vi "sub_saveData.vi"(8 "에러 입력(에러 없음)":errorcluster, 9 "파일명":string, 10 "저장경로":path, 11 "VISA 참조 번호 입력":refnum<visa-resource-name>) -> (0 "에러 출력":errorcluster, 3 "VISA 참조 번호 출력":refnum<visa-resource-name>)   [LabVIEW 2020]
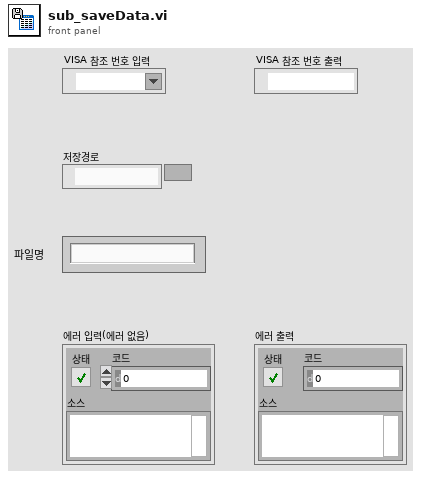
[diagram p1: front panel]
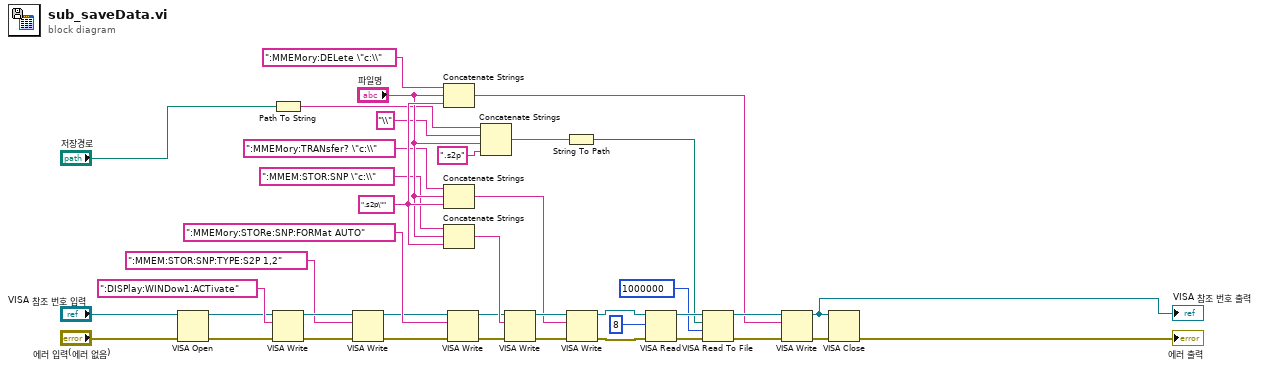
[diagram p0: block diagram]
diagram:
  w39 = ".s2p\"" ("문자열")
  n1 = VISA Open(error in (no error)="에러 입력(에러 없음)", VISA resource name="VISA 참조 번호 입력") -> (VISA resource name=w22:refnum<visa-resource-name>, error out=w23:errorcluster)  [unwired: 3 in]
  n2 = Path To String(path="저장경로") -> (string=w8:string)
  n3 = VISA Write(VISA resource name=w22, write buffer=":DISPlay:WINDow1:ACTivate" ("버퍼 쓰기"), error in (no error)=w23) -> (VISA resource name out=w24:refnum<visa-resource-name>, error out=w25:errorcluster)  [unwired: 1 out]
  n4 = VISA Write(VISA resource name=w24, write buffer=":MMEM:STOR:SNP:TYPE:S2P 1,2" ("버퍼 쓰기"), error in (no error)=w25) -> (VISA resource name out=w27:refnum<visa-resource-name>, error out=w28:errorcluster)  [unwired: 1 out]
  n5 = Concatenate Strings(":MMEMory:DELete \"c:\\" ("버퍼 쓰기"), "파일명", w39) -> (w3:string)
  n6 = Concatenate Strings(":MMEMory:TRANsfer? \"c:\\" ("버퍼 쓰기"), "파일명", w39) -> (w10:string)
  n7 = Concatenate Strings(":MMEM:STOR:SNP \"c:\\" ("버퍼 쓰기"), "파일명", w39) -> (w38:string)
  n8 = VISA Write(VISA resource name=w27, write buffer=":MMEMory:STORe:SNP:FORMat AUTO" ("버퍼 쓰기"), error in (no error)=w28) -> (VISA resource name out=w30:refnum<visa-resource-name>, error out=w34:errorcluster)  [unwired: 1 out]
  n9 = Concatenate Strings(w8, "\\" ("문자열"), "파일명", ".s2p" ("문자열")) -> (w7:string)
  n10 = VISA Write(VISA resource name=w30, write buffer=w38, error in (no error)=w34) -> (VISA resource name out=w31:refnum<visa-resource-name>, error out=w35:errorcluster)  [unwired: 1 out]
  n11 = String To Path(string=w7) -> (path=w6:path)
  n12 = VISA Write(VISA resource name=w31, write buffer=w10, error in (no error)=w35) -> (VISA resource name out=w33:refnum<visa-resource-name>, error out=w11:errorcluster)  [unwired: 1 out]
  n13 = VISA Read(VISA resource name=w33, byte count=u32 8 ("바이트 카운트"), error in (no error)=w11) -> (VISA resource name out=w32:refnum<visa-resource-name>, error out=w9:errorcluster)  [unwired: 2 out]
  n14 = VISA Read To File(8:w9, 9:u32 1000000 ("바이트 카운트"), 10:w6, 11:w32) -> (0:w4:errorcluster, 3:w5:refnum<visa-resource-name>)  [unwired: 1 out]
  n15 = VISA Write(VISA resource name=w5, write buffer=w3, error in (no error)=w4) -> (VISA resource name out=w40:refnum<visa-resource-name>, error out=w2:errorcluster)  [unwired: 1 out]
  "VISA 참조 번호 출력" <- w40
  n16 = VISA Close(VISA resource name=w40, error in (no error)=w2) -> (error out=→"에러 출력":errorcluster)
